vi "Load Parallel Subroutine.vi"(4 "Path Builder":refnum<class "IPath Builder.lvclass">, 5 "Parallel in":refnum<class "Parallel.lvclass">, 6 "Persistence in":refnum<class "IPersist.lvclass">, 7 "Linked List ID":string, 8 "error in (no error)":errorcluster, 10 "Paths":path[](array[path]), 11 "Linked List Ref":refnum<data-value>) -> (0 "error out":errorcluster, 3 "Linked List Ref out":refnum<data-value>)   [LabVIEW 2017]
uses:
  ITestExecutive/ITest Executive.lvclass
  linked-list/Source/Linked List/Linked List Ref/Linked List Ref.lvclass
  60a4713c-9991-498e-b8cc-026215c46d89.vi
  TestExecutive Ref/TestExecutive Ref.lvclass
  ebd35830-aab3-4a8c-9439-be88075cf000.vi
  07fadd7c-f439-428d-8b7d-a5d48cbb0b9a.vi
  807f29ff-2c0d-4845-96e3-26f7bacf8274.vi
  TestExecutive/Test Executive.lvclass
  0686657e-ce3c-4cb1-8915-926bffe558a0.vi
  8f5accf5-3a0b-49c7-8256-3e71f9fad646.vi
  350e5f9f-4912-4a60-9d4e-228846dd99f0.vi
  9afac329-2102-4699-842b-ef5eac783a5a.vi
  C:/Users/jonmc/Documents/Git/Test Executive/Source/Test Executive/ITestExecutive/ITest Executive.lvclass
  linked-list/Source/Linked List/ILinkedList/ILinked List.lvclass
  persistence/source/IPersist/IPersist.lvclass
  Path Builder/IPath Builder/IPath Builder.lvclass
  Parallel.lvclass
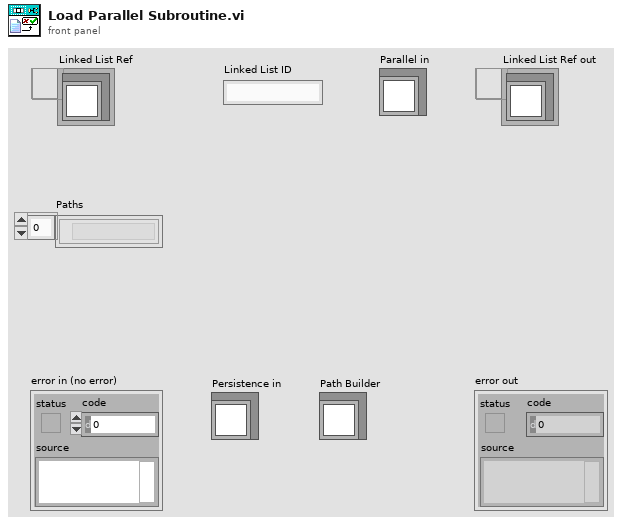
[diagram p1: front panel]
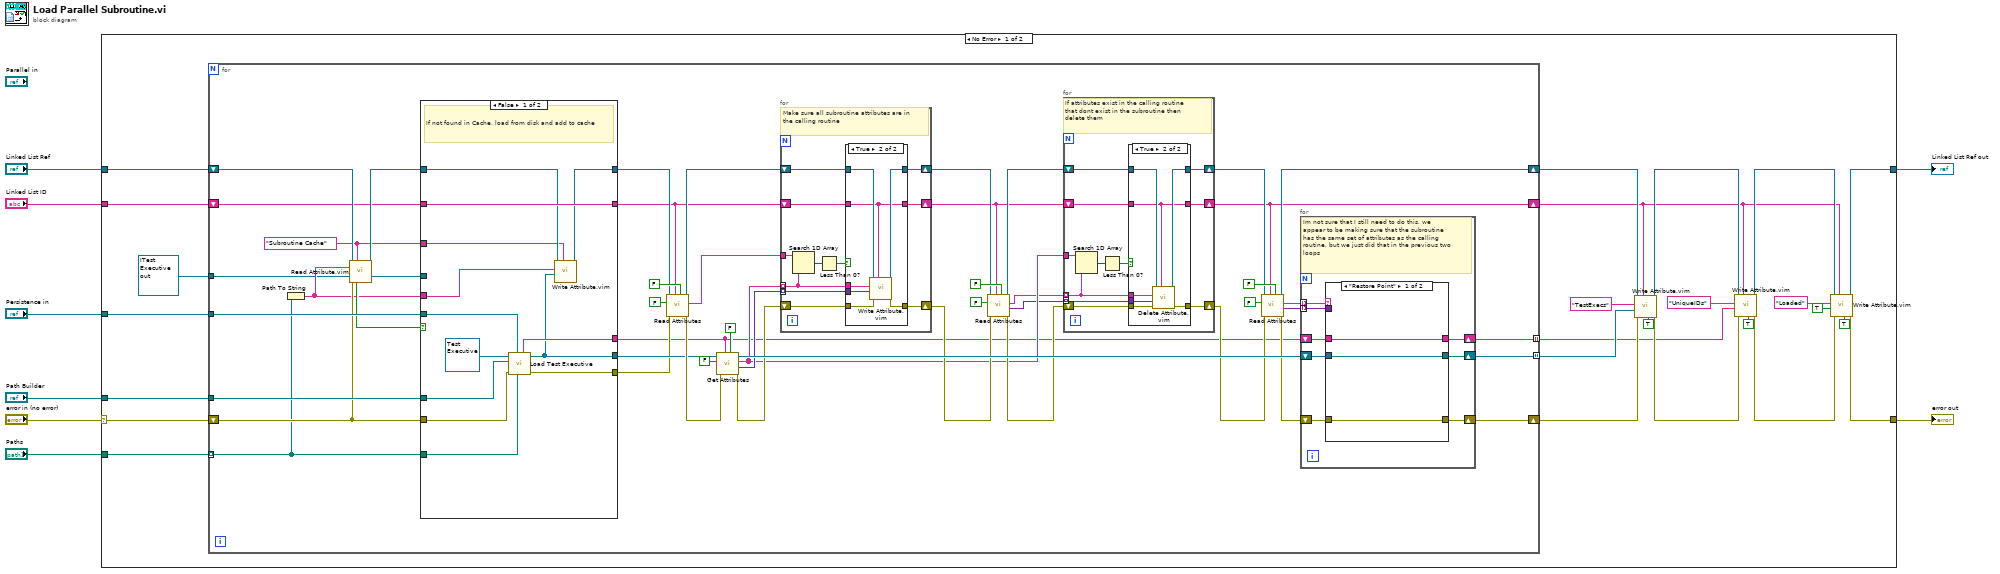
[diagram p0: block diagram]
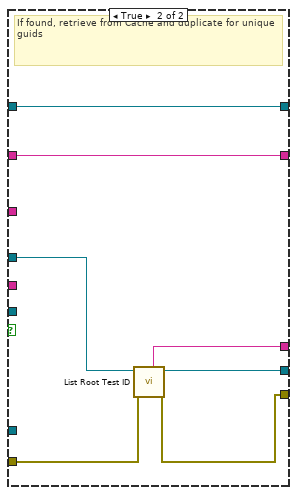
[diagram p2: hidden frame]
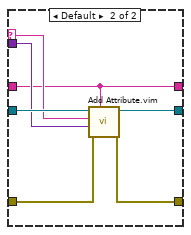
[diagram p5: hidden frame]
diagram:
  n1 = case shown="No Error" "error in (no error)" {
    selector: "error in (no error)" -> [w30 w163]
    tunnel: "Persistence in" -> [w33 _]
    tunnel: "Paths" -> [w29 _]
    tunnel: "Path Builder" -> [w32 _]
    tunnel: "Linked List Ref" -> [w31 w164]
    tunnel: "Linked List ID" -> [w28 _]
    tunnel: [w14 w164] -> w2
    tunnel: [w12 w163] -> w3
    frame No Error {
      n2 = for {
        tunnel: w33 -> [w82]
        tunnel: w32 -> [w81]
        tunnel: w29 -> [w51] mode=indexing
        tunnel: [w34] -> w9 mode=indexing
        shift-right: [w38] -> w15
        shift-left: w31 -> [w53]
        shift-right: [w37] -> w13
        shift-left: w30 -> [w52]
        shift-right: [w36] -> w11
        shift-left: w28 -> [w48]
        tunnel: refnum<data-value> refnum ("Test Executive Ref out") -> [w45]
        tunnel: [w35] -> w10 mode=indexing
        w46 = "Subroutine Cache" ("Name")
        n3 = Path To String(path=w51) -> (string=w47:string)
        n4 = call "Read Attribute.vim"("Linked List Ref"=w53, "Linked List ID"=w46, "Attribute Name"=w47, "Type"=w45, "error in (no error)"=w52) -> ("Linked List Ref out"=w49:refnum<data-value>, "Attribute"=w44:refnum<data-value>, "Found?"=w50:bool)  [unwired: 5 in, 3 out]
        n5 = case shown="False" w50 {
          tunnel: [w94 w99] -> w40
          tunnel: w82 -> [w93 _]
          tunnel: w81 -> [w92 _]
          tunnel: [w83 w97] -> w41
          tunnel: [w84 w96] -> w39
          tunnel: w52 -> [w91 w100]
          tunnel: w51 -> [w90 _]
          tunnel: [w87 w102] -> w43
          tunnel: w49 -> [w88 w102]
          tunnel: [w89 w101] -> w42
          tunnel: w48 -> [w89 w101]
          tunnel: w47 -> [w85 _]
          tunnel: w46 -> [w86 _]
          tunnel: w44 -> [_ w98]
          frame False {
            # "If not found in Cache, load from disk and add to cache"
            n6 = call "Load Test Executive.vi"("Folder"=w90, "Persistence in"=w93, "error in (no error)"=w91, "Path Builder"=w92, "Test Executive"=refnum<class "Test Executive.lvclass"> refnum ("Test Executive.lvlib:Test Executive.lvclass")) -> ("error out"=w94:errorcluster, "Test Executive Ref out"=w83:refnum<data-value>, "Root ID"=w84:string)  [unwired: 4 in]
            n7 = call "Write Attribute.vim"("Linked List ID"=w86, "Attribute"=w83, "Attribute Name"=w85, "Linked List Ref"=w88) -> ("Linked List Ref out"=w87:refnum<data-value>)  [unwired: 4 in, 3 out]
          }
          frame True {
            # "If found, retrieve from Cache and duplicate for unique guids"
            n8 = call "List Root Test ID.vi"("error in (no error)"=w100, "Test Executive Ref"=w98) -> ("error out"=w99:errorcluster, "Test Executive Ref out"=w97:refnum<data-value>, "Root ID"=w96:string)  [unwired: 5 in, 2 out]
          }
        }
        n9 = call "Read Attributes.vi"("Flatten Pointer?"=FALSE, "Linked List ID"=w42, "error in (no error)"=w40, "Include Private?"=FALSE, "Linked List Ref"=w43) -> ("error out"=w75:errorcluster, "Attribute Names out"=w74:string[], "Linked List Ref out"=w72:refnum<data-value>)  [unwired: 1 in, 3 out]
        n10 = call "Get Attributes.vi"("Flatten Pointer?"=FALSE, "Test ID"=w39, "error in (no error)"=w75, "Include Private?"=FALSE, "Test Executive Ref"=w41) -> ("error out"=w71:errorcluster, "Attributes"=w73:variant[], "Attribute Names out"=w63:string[], "Test Executive Ref out"=w78:refnum<data-value>)  [unwired: 1 in, 2 out]
        n11 = for {
          tunnel: w63 -> [w126] mode=indexing
          tunnel: w73 -> [w125] mode=indexing
          shift-right: [w131] -> w67
          shift-left: w72 -> [w132]
          tunnel: w74 -> [w133]
          shift-right: [w129] -> w68
          shift-left: w71 -> [w130]
          shift-right: [w124] -> w65
          shift-left: w42 -> [w128]
          # "Make sure all subroutine attributes are in the calling routine"
          n12 = Search 1D Array(1D array=w133, element=w126) -> (index of element=w134:i32)  [unwired: 1 in]
          n13 = Less Than 0?(x=w134) -> (x < 0?=w127:bool)
          n14 = case shown="True" w127 {
            tunnel: w132 -> [w137 w144]
            tunnel: [w137 w143] -> w131
            tunnel: w130 -> [w136 w142]
            tunnel: [w136 w141] -> w129
            tunnel: w128 -> [w135 w138]
            tunnel: w126 -> [_ w140]
            tunnel: w125 -> [_ w139]
            tunnel: [w135 w138] -> w124
            frame False {
            }
            frame True {
              n15 = call "Write Attribute.vim"("Linked List ID"=w138, "error in (no error)"=w142, "Attribute"=w139, "Attribute Name"=w140, "Linked List Ref"=w144) -> ("error out"=w141:errorcluster, "Linked List Ref out"=w143:refnum<data-value>)  [unwired: 3 in, 2 out]
            }
          }
        }
        n16 = call "Read Attributes.vi"("Flatten Pointer?"=FALSE, "Linked List ID"=w65, "error in (no error)"=w68, "Include Private?"=FALSE, "Linked List Ref"=w67) -> ("error out"=w64:errorcluster, "Attributes"=w61:variant[], "Attribute Names out"=w62:string[], "Linked List Ref out"=w66:refnum<data-value>)  [unwired: 1 in, 2 out]
        n17 = for {
          tunnel: w62 -> [w105] mode=indexing
          tunnel: w61 -> [w104] mode=indexing
          shift-right: [w110] -> w58
          shift-left: w66 -> [w111]
          tunnel: w63 -> [w112]
          shift-right: [w108] -> w57
          shift-left: w64 -> [w109]
          shift-right: [w103] -> w36
          shift-left: w65 -> [w107]
          # "If attributes exist in the calling routine that dont exist in the subroutine then delete them"
          n18 = Search 1D Array(1D array=w112, element=w105) -> (index of element=w113:i32)  [unwired: 1 in]
          n19 = Less Than 0?(x=w113) -> (x < 0?=w106:bool)
          n20 = case shown="True" w106 {
            tunnel: w111 -> [w116 w123]
            tunnel: [w116 w122] -> w110
            tunnel: w109 -> [w115 w120]
            tunnel: [w115 w119] -> w108
            tunnel: w107 -> [w114 w121]
            tunnel: w105 -> [_ w118]
            tunnel: w104 -> [_ w117]
            tunnel: [w114 w121] -> w103
            frame False {
            }
            frame True {
              n21 = call "Delete Attribute.vim"("Linked List ID"=w121, "error in (no error)"=w120, "Type"=w117, "Attribute Name"=w118, "Linked List Ref"=w123) -> ("error out"=w119:errorcluster, "Linked List Ref out"=w122:refnum<data-value>)  [unwired: 4 in, 1 out]
            }
          }
        }
        n22 = call "Read Attributes.vi"("Flatten Pointer?"=FALSE, "Linked List ID"=w36, "error in (no error)"=w57, "Include Private?"=FALSE, "Linked List Ref"=w58) -> ("error out"=w56:errorcluster, "Attributes"=w55:variant[], "Attribute Names out"=w54:string[], "Linked List Ref out"=w38:refnum<data-value>)  [unwired: 1 in, 2 out]
        n23 = for {
          shift-right: [w149] -> w37
          shift-left: w56 -> [w150]
          tunnel: w54 -> [w148] mode=indexing
          tunnel: w55 -> [w147] mode=indexing
          shift-right: [w146] -> w34
          shift-left: w39 -> [w151]
          shift-right: [w145] -> w35
          shift-left: w78 -> [w152]
          # "Im not sure that I still need to do this, we appear to be making sure that the subroutine has the same set of attributes as the calling routine, but we just did that in the previous two loops"
          n24 = case shown="\"Restore Point\"" w148 {
            selector: w148 -> [_ w159]
            tunnel: w152 -> [w153 w162]
            tunnel: w151 -> [w154 w157]
            tunnel: w150 -> [w155 w161]
            tunnel: [w155 w160] -> w149
            tunnel: w147 -> [_ w158]
            tunnel: [w154 w157] -> w146
            tunnel: [w153 w156] -> w145
            frame "Restore Point" {
            }
            frame Default {
              n25 = call "Add Attribute.vim"("ID"=w157, "error in (no error)"=w161, "Attribute"=w158, "Attribute Name"=w159, "Test Executive Ref"=w162) -> ("error out"=w160:errorcluster, "Test Executive Ref out"=w156:refnum<data-value>)  [unwired: 3 in, 2 out]
            }
          }
        }
      }
      n26 = call "Write Attribute.vim"("Private?"=TRUE, "Linked List ID"=w11, "error in (no error)"=w13, "Attribute"=w10, "Attribute Name"="TestExecs", "Linked List Ref"=w15) -> ("error out"=w23:errorcluster, "Linked List Ref out"=w17:refnum<data-value>)  [unwired: 2 in, 2 out]
      n27 = call "Write Attribute.vim"("Private?"=TRUE, "Linked List ID"=w11, "error in (no error)"=w23, "Attribute"=w9, "Attribute Name"="UniqueIDs", "Linked List Ref"=w17) -> ("error out"=w19:errorcluster, "Linked List Ref out"=w16:refnum<data-value>)  [unwired: 2 in, 2 out]
      n28 = call "Write Attribute.vim"("Private?"=TRUE, "Linked List ID"=w11, "error in (no error)"=w19, "Attribute"=TRUE, "Attribute Name"="Loaded", "Linked List Ref"=w16) -> ("error out"=w12:errorcluster, "Linked List Ref out"=w14:refnum<data-value>)  [unwired: 2 in, 2 out]
    }
    frame Error {
    }
  }
  "error out" <- w3
  "Linked List Ref out" <- w2
